vi "SystemController.ReftoDVR.vi"(10 "Ref":u32 format="%08x") -> (2 "Ref":T1)   [LabVIEW 2017, in "SystemController.lvclass"]
doc: "JKI State Machine Objects (SMO) 1.0.0.5\nJKI - JKI\nCopyright (c) 2016, JKI"
uses:
  SystemController.lvclass
  Typedefs/PrivateData--Ref.ctl
  Typedefs/PrivateData--Cluster.ctl
  Typedefs/Configuration--Cluster.ctl
  Typedefs/CameraConfig--Cluster.ctl
  Camera/Camera_IMAQdx_class/typedefs/Configuration--Cluster.ctl
  Typedefs/Dependencies--Cluster.ctl
  Camera/Camera_class/Camera.lvclass
  ImageFacialDetection_class/ImageFacialDetection.lvclass
  <vilib>/vision/Image Controls.llb/IMAQ Image.ctl
  Typedefs/PublicEvents--Cluster.ctl
  Typedefs/PublicEvents--SystemController.UIClosed.ctl
  Camera/Camera_IMAQdx_class/Camera_IMAQdx.lvclass
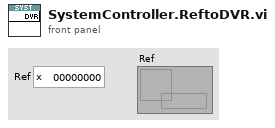
[diagram p1: front panel]
types:
  T1 = typedef "SystemController.lvclass/PrivateData--Ref.ctl" = refnum<data-value>
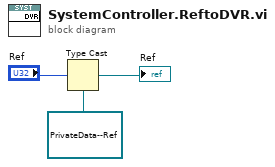
[diagram p0: block diagram]
diagram:
  n1 = Type Cast(type=T1 refnum ("Ref"), x="Ref") -> (*(type *) &x=→"Ref":T1)
